vi "getFile.vi"(7 "LabVIEW Web Service Request":refnum<class "Web Request.lvclass">, 11 "MAC":string) -> ()   [LabVIEW 2016]
uses:
  <vilib>/wsapi/Web Request.lvclass
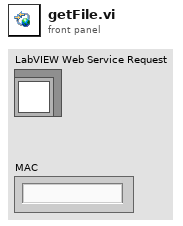
[diagram p1: front panel]
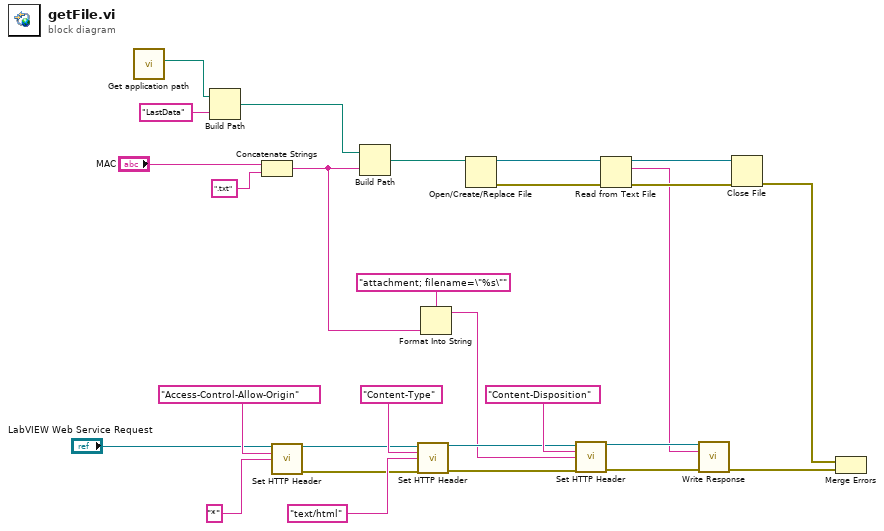
[diagram p0: block diagram]
diagram:
  n1 = call "Get application path.vi"() -> ("Application path"=w1:path)  [unwired: 11 in]
  n2 = Build Path(base path=w1, name or relative path="LastData") -> (appended path=w16:path)
  n3 = Concatenate Strings("MAC", ".txt" ("string")) -> (w13:string)
  n4 = call <vilib>:"Set HTTP Header.vi"("LabVIEW Web Service Request"="LabVIEW Web Service Request", "header"="Access-Control-Allow-Origin", "header value"="*") -> ("LabVIEW Web Service Request out"=w23:refnum<class "Web Request.lvclass">, "error out"=w20:errorcluster)  [unwired: 11 in]
  n5 = Build Path(base path=w16, name or relative path=w13) -> (appended path=w12:path)
  n6 = call <vilib>:"Set HTTP Header.vi"("LabVIEW Web Service Request"=w23, "header"="Content-Type", "header value"="text/html", "error in (no error)"=w20) -> ("LabVIEW Web Service Request out"=w21:refnum<class "Web Request.lvclass">, "error out"=w19:errorcluster)  [unwired: 10 in]
  n7 = Format Into String(format string="attachment; filename=\"%s\"", w13) -> (resulting string=w14:string)  [unwired: 2 in, 1 out]
  n8 = Open/Create/Replace File(file path (use dialog)=w12) -> (refnum out=w11:refnum<file>, error out=w10:errorcluster)  [unwired: 5 in, 1 out]
  n9 = call <vilib>:"Set HTTP Header.vi"("LabVIEW Web Service Request"=w21, "header"="Content-Disposition", "header value"=w14, "error in (no error)"=w19) -> ("LabVIEW Web Service Request out"=w7:refnum<class "Web Request.lvclass">, "error out"=w5:errorcluster)  [unwired: 10 in]
  n10 = Read from Text File(file (use dialog)=w11, error in=w10) -> (refnum out=w9:refnum<file>, text=w6:string, error out=w8:errorcluster)  [unwired: 2 in, 1 out]
  n11 = call <vilib>:"Write Response.vi"("LabVIEW Web Service Request"=w7, "response string"=w6, "error in (no error)"=w5) -> ("error out"=w4:errorcluster)  [unwired: 11 in, 1 out]
  n12 = Close File(refnum=w9, error in=w8) -> (error out=w3:errorcluster)  [unwired: 1 out]
  n13 = Merge Errors(w3, w4) -> ()  [unwired: 1 out]
